vi "Draw XY Data.vi"(4 "[sized scatter plot cosmetics]":T1={"min size"=1, "max size"=5, "maps to max size"=5, "color array"=[16776960, 65280, 16711680, 255]}, 6 "xy cosmetics":T3={"plot color"=16776960, "plot type"=enum."connected points", "baseline"=0.0} {"baseline" format="%0.2f"}, 8 "xy data":cluster{"x":dbl, "y":dbl}[](array[cluster]) {"y" format="%0.2f"; "x" format="%0.2f"}, 9 "y scale factors":cluster{"a":dbl, "b":dbl, "log?":bool} {"b" format="%0.2f"; "a" format="%0.2f"}, 10 "x scale factors":cluster{"a":dbl, "b":dbl, "log?":bool} {"b" format="%0.2f"; "a" format="%0.2f"}, 11 "picture":picture) -> (3 "new picture":picture)   [LabVIEW 2012, in "Vector Function Generator.xctl"]
doc: "Original version modified by G. Burnell (g.burnell@leeds.ac.uk) for plotting on black background."
uses:
  Vector Function Generator.xctl
  <vilib>/picture/cartesn2.llb/XY Plot Type.ctl
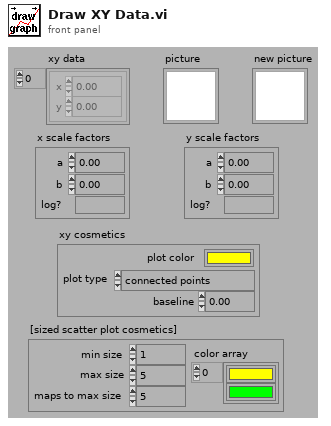
[diagram p1: front panel]
types:
  T1 = cluster{"min size":i16, "max size":i16, "maps to max size":i16, "color array":u32[]}
  T2 = typedef "XY Plot Type.ctl" = enum16{"points", "squares", "circles", "connected points", "connected squares", "connected circles", "comb plot", "sized scatter plot", "sized-colored scatter plot", "min-max lines"}
  T3 = cluster{"plot color":u32, "plot type":T2, "baseline":dbl}
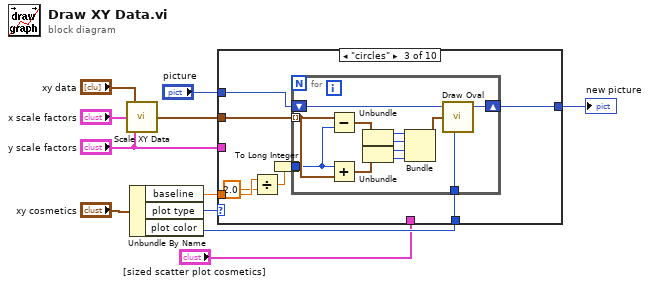
[diagram p0: block diagram]
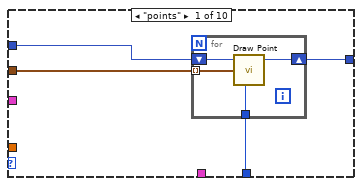
[diagram p2: hidden frame]
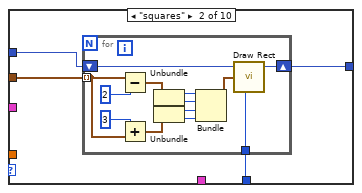
[diagram p3: hidden frame]
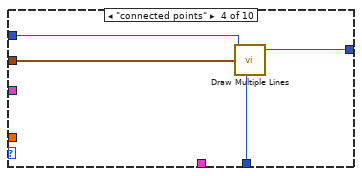
[diagram p4: hidden frame]
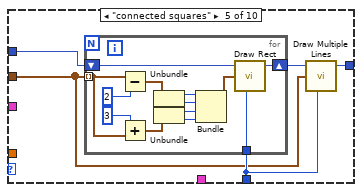
[diagram p5: hidden frame]
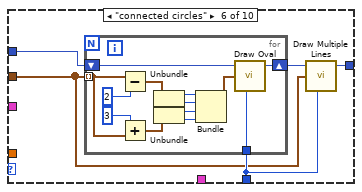
[diagram p6: hidden frame]
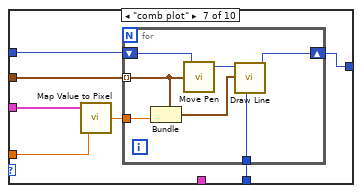
[diagram p7: hidden frame]
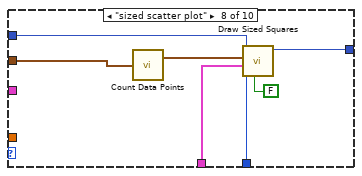
[diagram p8: hidden frame]
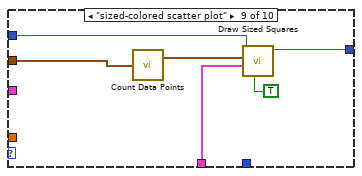
[diagram p9: hidden frame]
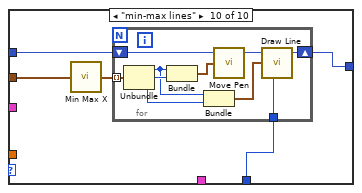
[diagram p10: hidden frame]
diagram:
  n1 = call <vilib>:"Scale XY Data.vi"("y scale factors"="y scale factors", "x scale factors"="x scale factors", "xy data"="xy data") -> ("scaled xy data"=w8:cluster{"x":i16, "y":i16}[])
  n2 = Unbundle By Name("xy cosmetics") -> ("baseline"=w3:dbl, "plot type"=w4:T2, "plot color"=w11:u32)
  n3 = case shown="\"circles\"" w4 {
    tunnel: w11 -> [w15 w20 w41 w59 w65 w83 w97 w113 _ w127]
    tunnel: [w14 w21 w42 w60 w63 w81 w100 w117 w120 w124] -> w10
    tunnel: "picture" -> [w13 w22 w43 w57 w62 w80 w101 w114 w122 w128]
    tunnel: w8 -> [w12 w23 w44 w58 w61 w79 w99 w115 w123 w125]
    tunnel: w3 -> [_ _ w40 _ _ _ w102 _ _ _]
    tunnel: "y scale factors" -> [_ _ _ _ _ _ w103 _ _ _]
    tunnel: "[sized scatter plot cosmetics]" -> [_ _ _ _ _ _ _ w112 w119 _]
    frame "points" {
      n4 = for {
        shift-right: [w19] -> w14
        shift-left: w13 -> [w18]
        tunnel: w15 -> [w17]
        tunnel: w12 -> [w16] mode=indexing
        n5 = call <vilib>:"Draw Point.vi"("picture"=w18, "point(x,y)"=w16, "color(black)"=w17) -> ("new picture"=w19:picture)  [unwired: 1 in, 5 out]
      }
    }
    frame "squares" {
      n6 = for {
        tunnel: w23 -> [w33] mode=indexing
        shift-right: [w36] -> w21
        shift-left: w22 -> [w35]
        tunnel: w20 -> [w34]
        n7 = Subtract(x=w33, y=i16 2) -> (x-y=w26:cluster{"x":i16, "y":i16})
        n8 = Add(x=i16 3, y=w33) -> (x+y=w32:cluster{"x":i16, "y":i16})
        n9 = Unbundle(w26) -> ("x"=w28:i16, "y"=w29:i16)
        n10 = Unbundle(w32) -> ("x"=w30:i16, "y"=w31:i16)
        n11 = Bundle("x"=w28, "y"=w29, "x"=w30, "y"=w31) -> (w27:cluster{"x":i16, "y":i16, "x":i16, "y":i16})  [unwired: 1 out]
        n12 = call <vilib>:"Draw Rect.vi"("picture"=w35, "rect"=w27, "color(black)"=w34) -> ("new picture"=w36:picture)  [unwired: 2 in, 4 out]
      }
    }
    frame "circles" {
      n13 = Divide(x=w40, y=2.0) -> (x/y=w38:dbl)
      n14 = To Long Integer(number=w38) -> (32bit integer=w37:i32)
      n15 = for {
        tunnel: w44 -> [w53] mode=indexing
        shift-right: [w56] -> w42
        shift-left: w43 -> [w55]
        tunnel: w41 -> [w54]
        tunnel: w37 -> [w45]
        n16 = Subtract(x=w53, y=w45) -> (x-y=w46:cluster{"x":i32, "y":i32})
        n17 = Add(x=w45, y=w53) -> (x+y=w52:cluster{"x":i32, "y":i32})
        n18 = Unbundle(w46) -> ("x"=w48:i32, "y"=w49:i32)
        n19 = Unbundle(w52) -> ("x"=w50:i32, "y"=w51:i32)
        n20 = Bundle("x"=w48, "y"=w49, "x"=w50, "y"=w51) -> (w47:cluster{"x":i32, "y":i32, "x":i32, "y":i32})  [unwired: 1 out]
        n21 = call <vilib>:"Draw Oval.vi"("picture"=w55, "rect"=w47, "color(black)"=w54) -> ("new picture"=w56:picture)  [unwired: 2 in, 4 out]
      }
    }
    frame "connected points" {
      n22 = call <vilib>:"Draw Multiple Lines.vi"("picture"=w57, "line endpoints"=w58, "color(black)"=w59) -> ("new picture"=w60:picture)  [unwired: 2 in, 4 out]
    }
    frame "connected squares" {
      n23 = for {
        tunnel: w61 -> [w69] mode=indexing
        shift-right: [w78] -> w64
        shift-left: w62 -> [w77]
        tunnel: w65 -> [w71]
        n24 = Subtract(x=w69, y=i16 2) -> (x-y=w68:cluster{"x":i16, "y":i16})
        n25 = Add(x=i16 3, y=w69) -> (x+y=w70:cluster{"x":i16, "y":i16})
        n26 = Unbundle(w68) -> ("x"=w76:i16, "y"=w75:i16)
        n27 = Unbundle(w70) -> ("x"=w74:i16, "y"=w73:i16)
        n28 = Bundle("x"=w76, "y"=w75, "x"=w74, "y"=w73) -> (w72:cluster{"x":i16, "y":i16, "x":i16, "y":i16})  [unwired: 1 out]
        n29 = call <vilib>:"Draw Rect.vi"("picture"=w77, "rect"=w72, "color(black)"=w71) -> ("new picture"=w78:picture)  [unwired: 2 in, 4 out]
      }
      n30 = call <vilib>:"Draw Multiple Lines.vi"("picture"=w64, "line endpoints"=w61, "color(black)"=w65) -> ("new picture"=w63:picture)  [unwired: 2 in, 4 out]
    }
    frame "connected circles" {
      n31 = for {
        tunnel: w79 -> [w87] mode=indexing
        shift-right: [w96] -> w82
        shift-left: w80 -> [w95]
        tunnel: w83 -> [w89]
        n32 = Subtract(x=w87, y=i16 2) -> (x-y=w86:cluster{"x":i16, "y":i16})
        n33 = Add(x=i16 3, y=w87) -> (x+y=w88:cluster{"x":i16, "y":i16})
        n34 = Unbundle(w86) -> ("x"=w94:i16, "y"=w93:i16)
        n35 = Unbundle(w88) -> ("x"=w92:i16, "y"=w91:i16)
        n36 = Bundle("x"=w94, "y"=w93, "x"=w92, "y"=w91) -> (w90:cluster{"x":i16, "y":i16, "x":i16, "y":i16})  [unwired: 1 out]
        n37 = call <vilib>:"Draw Oval.vi"("picture"=w95, "rect"=w90, "color(black)"=w89) -> ("new picture"=w96:picture)  [unwired: 2 in, 4 out]
      }
      n38 = call <vilib>:"Draw Multiple Lines.vi"("picture"=w82, "line endpoints"=w79, "color(black)"=w83) -> ("new picture"=w81:picture)  [unwired: 2 in, 4 out]
    }
    frame "comb plot" {
      n39 = call <vilib>:"Map Value to Pixel.vi"("x"=w102, "scale factors"=w103) -> ("pixel"=w98:dbl)  [unwired: 1 out]
      n40 = for {
        shift-right: [w108] -> w100
        shift-left: w101 -> [w110]
        tunnel: w99 -> [w106] mode=indexing
        tunnel: w98 -> [w107]
        tunnel: w97 -> [w104]
        n41 = Bundle(cluster=w106, "y"=w107) -> (w105:cluster{"x":i16, "y":i16})  [unwired: 1 out]
        n42 = call <vilib>:"Move Pen.vi"("new position"=w106, "picture"=w110) -> ("new picture"=w109:picture)  [unwired: 1 in, 2 out]
        n43 = call <vilib>:"Draw Line.vi"("picture"=w109, "end point"=w105, "color(black)"=w104) -> ("new picture"=w108:picture)  [unwired: 2 in, 4 out]
      }
    }
    frame "sized scatter plot" {
      n44 = call <vilib>:"Count Data Points.vi"("scaled xy data"=w115) -> ("counted data"=w116:cluster{"x":i16, "y":i16, "c":i16}[])  [unwired: 1 out]
      n45 = call <vilib>:"Draw Sized Squares.vi"("multi-color(F)"=FALSE, "color(yellow)"=w113, "sized scatter plot cosmetics"=w112, "data"=w116, "picture"=w114) -> ("new picture"=w117:picture)  [unwired: 6 out]
    }
    frame "sized-colored scatter plot" {
      n46 = call <vilib>:"Count Data Points.vi"("scaled xy data"=w123) -> ("counted data"=w121:cluster{"x":i16, "y":i16, "c":i16}[])  [unwired: 1 out]
      n47 = call <vilib>:"Draw Sized Squares.vi"("multi-color(F)"=TRUE, "sized scatter plot cosmetics"=w119, "data"=w121, "picture"=w122) -> ("new picture"=w120:picture)  [unwired: 1 in, 6 out]
    }
    frame "min-max lines" {
      n48 = call <vilib>:"Min Max X.vi"("scaled xy data"=w125) -> ("min max data"=w126:cluster{"x":i16, "min":i16, "max":i16}[])
      n49 = for {
        shift-right: [w138] -> w124
        shift-left: w128 -> [w135]
        tunnel: w126 -> [w134] mode=indexing
        tunnel: w127 -> [w137]
        n50 = Unbundle(w134) -> ("x"=w130:i16, "min"=w132:i16, "max"=w131:i16)
        n51 = Bundle("x"=w130, "min"=w132) -> (w129:cluster{"x":i16, "min":i16})  [unwired: 1 out]
        n52 = Bundle("x"=w130, "max"=w131) -> (w133:cluster{"x":i16, "max":i16})  [unwired: 1 out]
        n53 = call <vilib>:"Move Pen.vi"("new position"=w129, "picture"=w135) -> ("new picture"=w136:picture)  [unwired: 1 in, 2 out]
        n54 = call <vilib>:"Draw Line.vi"("picture"=w136, "end point"=w133, "color(black)"=w137) -> ("new picture"=w138:picture)  [unwired: 2 in, 4 out]
      }
    }
  }
  "new picture" <- w10
